vi "ValidacaoOndaContinua.vi"(11 "InfoContinuo":T1={"TempRampas"=0.0, "PicoMax"=0.0, "TextUnidMed"="segundos"}) -> (0 "error out":errorcluster)   [LabVIEW 2019]
uses:
  TelaConfig/Configuracao.Variaveis.vi
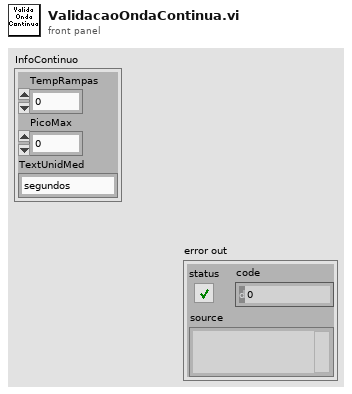
[diagram p1: front panel]
types:
  T1 = cluster{"TempRampas":dbl, "PicoMax":dbl, "TextUnidMed":string}
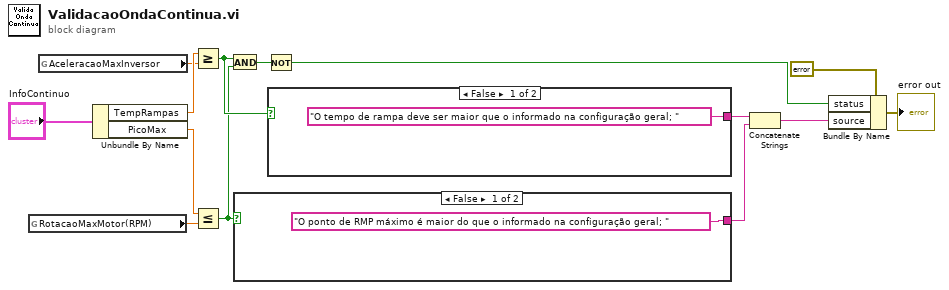
[diagram p0: block diagram]
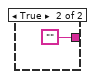
[diagram p2: hidden frame]
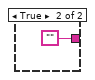
[diagram p3: hidden frame]
diagram:
  n1 = global read "Configuracao.Variaveis.vi" "RotacaoMaxMotor(RPM)"() -> (w11:dbl)
  n2 = global read "Configuracao.Variaveis.vi" "AceleracaoMaxInversor"() -> (w13:dbl)
  n3 = Unbundle By Name("InfoContinuo") -> ("TempRampas"=w14:dbl, "PicoMax"=w12:dbl)
  n4 = Greater Or Equal?(x=w14, y=w13) -> (x >= y?=w9:bool)
  n5 = Less Or Equal?(x=w12, y=w11) -> (x <= y?=w8:bool)
  n6 = And(x=w9, y=w8) -> (x .and. y?=w7:bool)
  n7 = case shown="False" w8 {
    tunnel: ["O ponto de RMP máximo é maior do que o informado na configuração geral; " ""] -> w2
    frame False {
    }
    frame True {
    }
  }
  n8 = Not(x=w7) -> (.not. x?=w4:bool)
  n9 = case shown="False" w9 {
    tunnel: ["O tempo de rampa deve ser maior que o informado na configuração geral; " ""] -> w3
    frame False {
    }
    frame True {
    }
  }
  n10 = Concatenate Strings(w3, w2) -> (w1:string)
  n11 = Bundle By Name(cluster=errorcluster {"status"=FALSE, "code"=0, "source"=""} ("error out"), "status"=w4, "source"=w1) -> (→"error out":errorcluster)
